vi "Pre-Build Action.vi"(6 "Top Level/Always Included VIs":path[](array[path]), 7 "Main Destination Path":path, 9 "Target Name":string, 10 "Build Specification Name":string, 11 "Project Path":path) -> (0 "error out":errorcluster)   [LabVIEW 2014]
uses:
  <vilib>/addons/_JKI Toolkits/Caraya/classes/Test Suite/Test Suite.lvclass
panel:
  out "TDD Results Log Path":path
  out "TDD Results":string
  # "Debug indicators - do not wire to conn pane!"
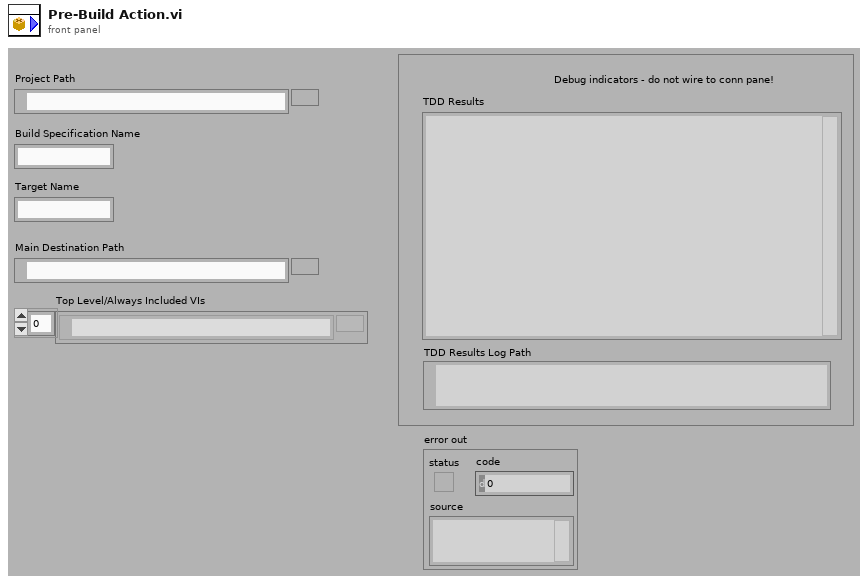
[diagram p1: front panel]
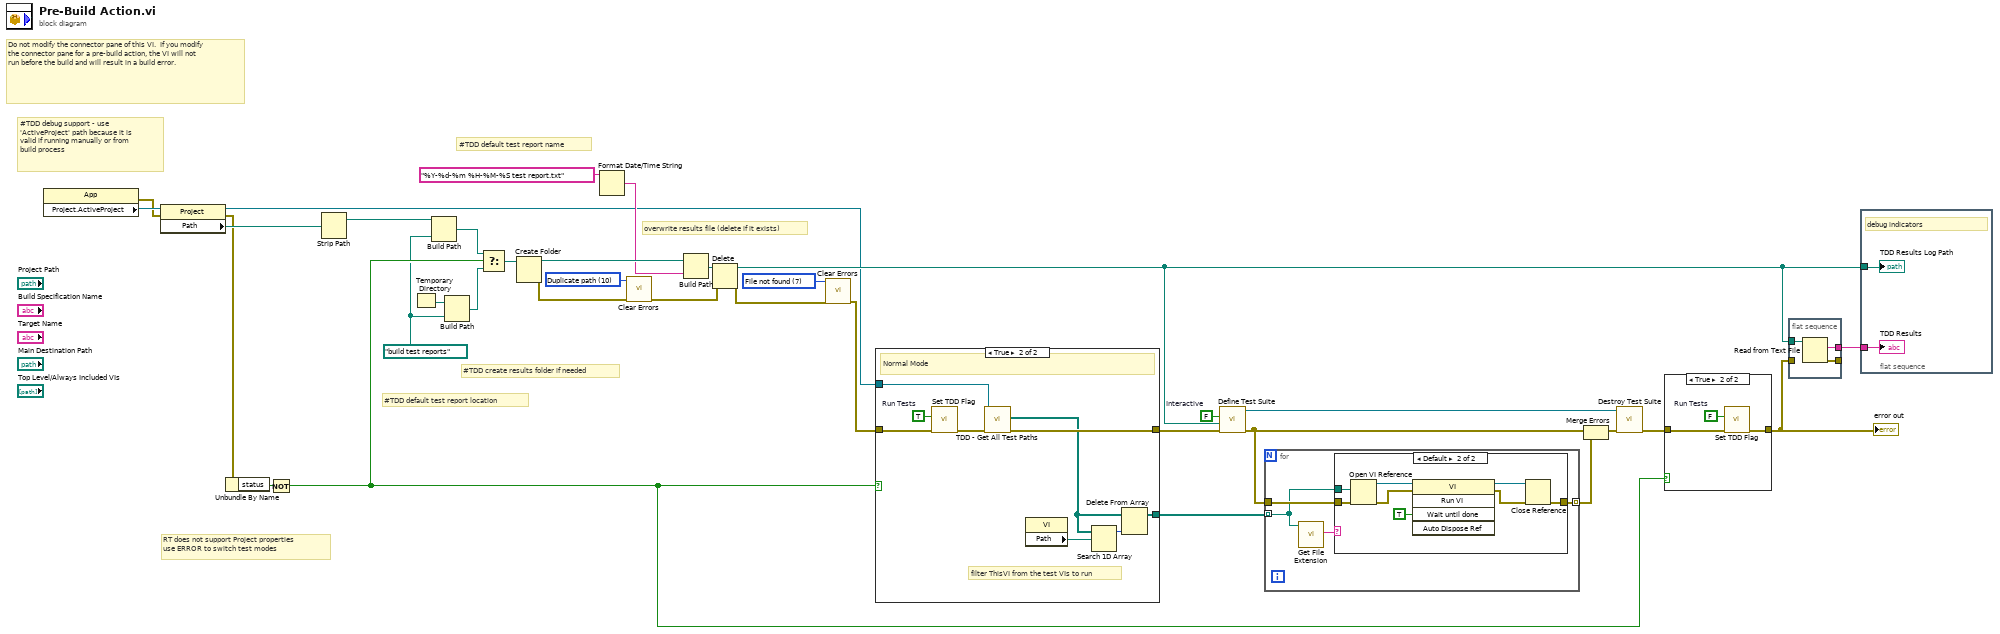
[diagram p0: block diagram]
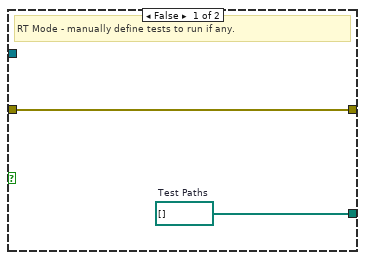
[diagram p3: hidden frame]
diagram:
  w13 = 7 items=["No error", "Argument error", "Memory is full", "Out of zone", "End of file", "File already open", "Generic file I/O error", "File not found", "File permission error", "Disk is full", "Duplicate path", "Too many files open", "System feature not enabled", "Resource file not found", "Cannot add resource", "Resource not found", "Image not found", "Image memory error", "Pen does not exist", "Config type invalid", "Config token not found", "Config parse error", "Config memory error", "Bad external code format", "Bad external code offset", "External code not present", "Null window", "Destroy window error", "Null menu", "Print aborted", "Bad print record", "Print driver error", "Windows error during printing", "Memory error during printing", "Print dialog error", "Generic print error", "Invalid device refnum", "Device not found", "Device parameter error", "Device unit error", "Cannot open device", "Device call aborted", "Generic error", "Cancelled by user", "Object ID too low", "Object ID too high", "Object not in heap", "Unknown heap", "Unknown object (invalid DefProc)", "Unknown object (DefProc not in table)", "Message out of range", "Invalid (null) method", "Unknown message", "Manager call not supported", "Bad address", "Network operation in progress", "Network operation timed out", "Connection is busy", "Network attribute not supported", "Network error", "Address in use", "System out of memory", "Connection aborted", "Connection refused", "Not connected", "Already connected", "Connection closed", "Initialization error (interapplication manager)", "Bad occurrence", "Wait on unbound occurrence handler", "Occurrence queue overflow", "Datalog type conflict", "Unused", "Unrecognized type (interapplication manager)", "Memory corrupt", "Failed to make temporary DLL", "Old CIN version", "Drag socket not found", "Failed to load drop-object", "Failed to register OLE object", "Failed to release OLE object", "Format specifier type mismatch", "Unknown format specifier", "Too few format specifiers", "Too many format specifiers", "Scan failed", "Newer CIN version", "Error converting to variant", "Runtime menu error", "Password tampered", "Variant attribute not found", "Incompatible variant data type", "Event data is not available", "Event Store is not present", "Occurrence is not found", "Event Queue is not created", "Event info is not available", "Refnum passed is NULL", "Error retrieving Class GUID", "Error retrieving CoClass GUID", "Error retrieving TypeLib GUID.", "Bad built application magic bytes.", "Specific driver is different from the specific driver associated with the Logical Name.", "There is no session opened to the class driver.", "Max Error", "MAX - Error with config objects", "MAX - Error loading configuration", "MAX - Group not supported"]
  w5 = path "build test reports" ("Report Path")
  w24 = 10 items=["No error", "Argument error", "Memory is full", "Out of zone", "End of file", "File already open", "Generic file I/O error", "File not found", "File permission error", "Disk is full", "Duplicate path", "Too many files open", "System feature not enabled", "Resource file not found", "Cannot add resource", "Resource not found", "Image not found", "Image memory error", "Pen does not exist", "Config type invalid", "Config token not found", "Config parse error", "Config memory error", "Bad external code format", "Bad external code offset", "External code not present", "Null window", "Destroy window error", "Null menu", "Print aborted", "Bad print record", "Print driver error", "Windows error during printing", "Memory error during printing", "Print dialog error", "Generic print error", "Invalid device refnum", "Device not found", "Device parameter error", "Device unit error", "Cannot open device", "Device call aborted", "Generic error", "Cancelled by user", "Object ID too low", "Object ID too high", "Object not in heap", "Unknown heap", "Unknown object (invalid DefProc)", "Unknown object (DefProc not in table)", "Message out of range", "Invalid (null) method", "Unknown message", "Manager call not supported", "Bad address", "Network operation in progress", "Network operation timed out", "Connection is busy", "Network attribute not supported", "Network error", "Address in use", "System out of memory", "Connection aborted", "Connection refused", "Not connected", "Already connected", "Connection closed", "Initialization error (interapplication manager)", "Bad occurrence", "Wait on unbound occurrence handler", "Occurrence queue overflow", "Datalog type conflict", "Unused", "Unrecognized type (interapplication manager)", "Memory corrupt", "Failed to make temporary DLL", "Old CIN version", "Drag socket not found", "Failed to load drop-object", "Failed to register OLE object", "Failed to release OLE object", "Format specifier type mismatch", "Unknown format specifier", "Too few format specifiers", "Too many format specifiers", "Scan failed", "Newer CIN version", "Error converting to variant", "Runtime menu error", "Password tampered", "Variant attribute not found", "Incompatible variant data type", "Event data is not available", "Event Store is not present", "Occurrence is not found", "Event Queue is not created", "Event info is not available", "Refnum passed is NULL", "Error retrieving Class GUID", "Error retrieving CoClass GUID", "Error retrieving TypeLib GUID.", "Bad built application magic bytes.", "Specific driver is different from the specific driver associated with the Logical Name.", "There is no session opened to the class driver.", "Max Error", "MAX - Error with config objects", "MAX - Error loading configuration", "MAX - Group not supported"]
  w30 = FALSE  # Interactive
  # "#TDD default test report location"
  # "RT does not support Project properties\nuse ERROR to switch test modes"
  # "#TDD create results folder if needed"
  # "overwrite results file (delete if it exists)"
  # "#TDD default test report name"
  # "#TDD debug support - use 'ActiveProject' path because it is valid if running manually or from build process"
  # "Do not modify the connector pane of this VI.  If you modify the connector pane for a pre-build action, the VI will not run before the build and will result in a build error."
  n1 = property class="App"() -> (error out=w3:errorcluster, "Project.ActiveProject"=w34:refnum<vi>)  [unwired: 2 in, 1 out]
  n2 = property class="Project"(reference=w34, error in=w3) -> (reference out=w1:refnum<vi>, error out=w2:errorcluster, "Path"=w7:path)
  n3 = Unbundle By Name(w2) -> ("status"=w19:bool)
  n4 = Not(x=w19) -> (.not. x?=w18:bool)
  n5 = Strip Path(path=w7) -> (stripped path=w6:path)  [unwired: 1 out]
  n6 = Temporary Directory() -> (w10:path)
  n7 = Build Path(base path=w6, name or relative path=w5) -> (appended path=w4:path)
  n8 = Build Path(base path=w10, name or relative path=w5) -> (appended path=w9:path)
  n9 = Select(t=w4, s=w18, f=w9) -> (s? t:f=w8:path)
  n10 = Create Folder(path (use dialog)=w8) -> (created path=w26:path, error out=w15:errorcluster)  [unwired: 2 in, 1 out]
  n11 = Format Date/Time String(time format string (%c)="%Y-%d-%m %H-%M-%S test report.txt") -> (date/time string=w25:string)  [unwired: 2 in]
  n12 = call <vilib>:"Clear Errors.vi"("error in (no error)"=w15, "specific error code to clear (0: all)"=w24) -> ("error out"=w14:errorcluster)  [unwired: 4 in, 1 out]
  n13 = Build Path(base path=w26, name or relative path=w25) -> (appended path=w20:path)
  n14 = Delete(path (use dialog)=w20, error in=w14) -> (deleted path=w31:path, error out=w12:errorcluster)  [unwired: 3 in, 1 out]
  n15 = call <vilib>:"Clear Errors.vi"("error in (no error)"=w12, "specific error code to clear (0: all)"=w13) -> ("error out"=w11:errorcluster)  [unwired: 4 in, 1 out]
  n16 = case shown="True" w18 {
    tunnel: w11 -> [w36 w45]
    tunnel: [w36 w40] -> w17
    tunnel: w1 -> [_ w38]
    tunnel: [w35 w37] -> w16
    frame False {
      w35 = path[] []  # Test Paths
      # "RT Mode - manually define tests to run if any."
    }
    frame True {
      w44 = TRUE  # Run Tests
      # "filter ThisVI from the test VIs to run"
      # "Normal Mode"
      n17 = call "Set TDD Flag.vi"("error in"=w45, "TDD Mode (T=Run Tests)"=w44) -> ("error out"=w41:errorcluster)  [unwired: 9 in]
      n18 = call "TDD - Get All Test Paths.vi"("error in (no error)"=w41, "Project in"=w38) -> ("error out"=w40:errorcluster, "Test Paths"=w39:path[])  [unwired: 8 in]
      n19 = property class="VI"() -> ("Path"=w42:path)  [unwired: 2 in, 2 out]
      n20 = Search 1D Array(1D array=w39, element=w42) -> (index of element=w43:i32)  [unwired: 1 in]
      n21 = Delete From Array(array=w39, index=w43) -> (array with subset deleted=w37:path[])  [unwired: 1 in, 1 out]
    }
  }
  n22 = call <vilib>:"Define Test Suite.vi"("error in (no error)"=w17, "Report Path"=w31, "Interactive"=w30) -> ("error out"=w22:errorcluster, "Test Suite"=w28:refnum<class "Test Suite.lvclass">)  [unwired: 7 in]
  n23 = for {
    tunnel: w22 -> [w48]
    tunnel: [w49] -> w29 mode=indexing
    tunnel: w16 -> [w47] mode=indexing
    n24 = call <vilib>:"Get File Extension.vi"("file"=w47) -> ("lowercase file extension"=w46:string)  [unwired: 7 in, 3 out]
    n25 = case shown="Default" w46 {
      tunnel: [w50 w53] -> w49
      tunnel: w48 -> [w50 w52]
      tunnel: w47 -> [_ w51]
      frame "vit" {
        # "do not run VI Templates as tests"
      }
      frame Default {
        n26 = Open VI Reference(vi path=w51, error in (no error)=w52) -> (vi reference=w57:refnum<vi>, error out=w55:errorcluster)  [unwired: 4 in]
        n27 = invoke class="VI" method="Run VI"(reference=w57, error in=w55, "Wait until done"=TRUE ("Wait Until Done")) -> (reference out=w56:refnum<vi>, error out=w54:errorcluster)  [unwired: 2 in, 3 out]
        n28 = Close Reference(reference=w56, error in (no error)=w54) -> (error out=w53:errorcluster)
      }
    }
  }
  n29 = Merge Errors(w22, w29) -> (w23:errorcluster)
  n30 = call-dynamic "Destroy Test Suite.vi"("error in (no error)"=w23, "Test Suite in"=w28) -> ("error out"=w21:errorcluster)  [unwired: 9 in]
  n31 = case shown="True" w18 {
    tunnel: [w59 w62] -> w33
    tunnel: w21 -> [w59 w61]
    frame False {
    }
    frame True {
      w60 = FALSE  # Run Tests
      n32 = call "Set TDD Flag.vi"("error in"=w61, "TDD Mode (T=Run Tests)"=w60) -> ("error out"=w62:errorcluster)  [unwired: 9 in]
    }
  }
  "error out" <- w33
  n33 = flat-sequence {
    tunnel: w33 -> [_]
    tunnel: w31 -> [w65]
    tunnel: [w64] -> w32
    tunnel: [w63] -> _
    frame #0 {
      n34 = Read from Text File(file (use dialog)=w65) -> (text=w64:string, error out=w63:errorcluster)  [unwired: 3 in, 2 out]
    }
  }
  n35 = flat-sequence {
    tunnel: w32 -> [w67]
    tunnel: w31 -> [w66]
    frame #0 {
      # "debug indicators"
      "TDD Results" <- w67
      "TDD Results Log Path" <- w66
    }
  }
